vi "TIFF_writeMultipage.vi"(8 "error in":errorcluster, 10 "Array in":T1[](array[typedef]), 11 "file (use dialog)":path=path "D:/TestLV3.tif") -> (0 "error out":errorcluster)   [LabVIEW 2019]
doc: "This VI writes an image array to a multipage tif file. Valid formats are U8 or U16."
uses:
  <vilib>/vision/Image Controls.llb/IMAQ Image.ctl
panel:
  out "First page":T1(plugin-control)
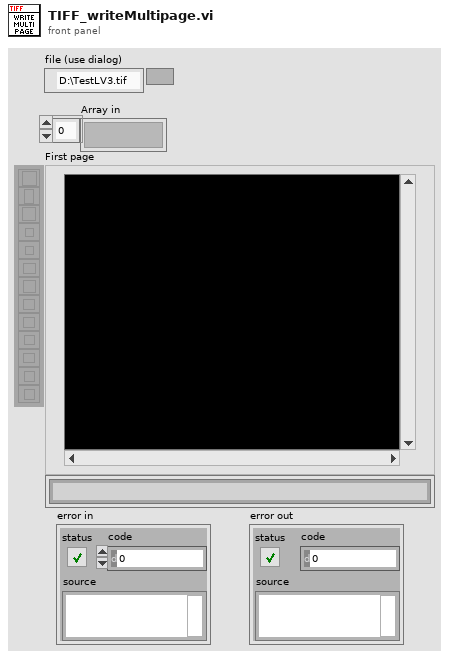
[diagram p1: front panel]
types:
  T1 = typedef "IMAQ Image.ctl" = refnum<image>
  T2 = enum16{"open", "replace", "create", "open or create", "replace or create", "replace or create with confirmation"}
  T3 = enum16{"big-endian, network order", "native, host order", "little-endian"}
  T4 = typedef "Image Type" = u32
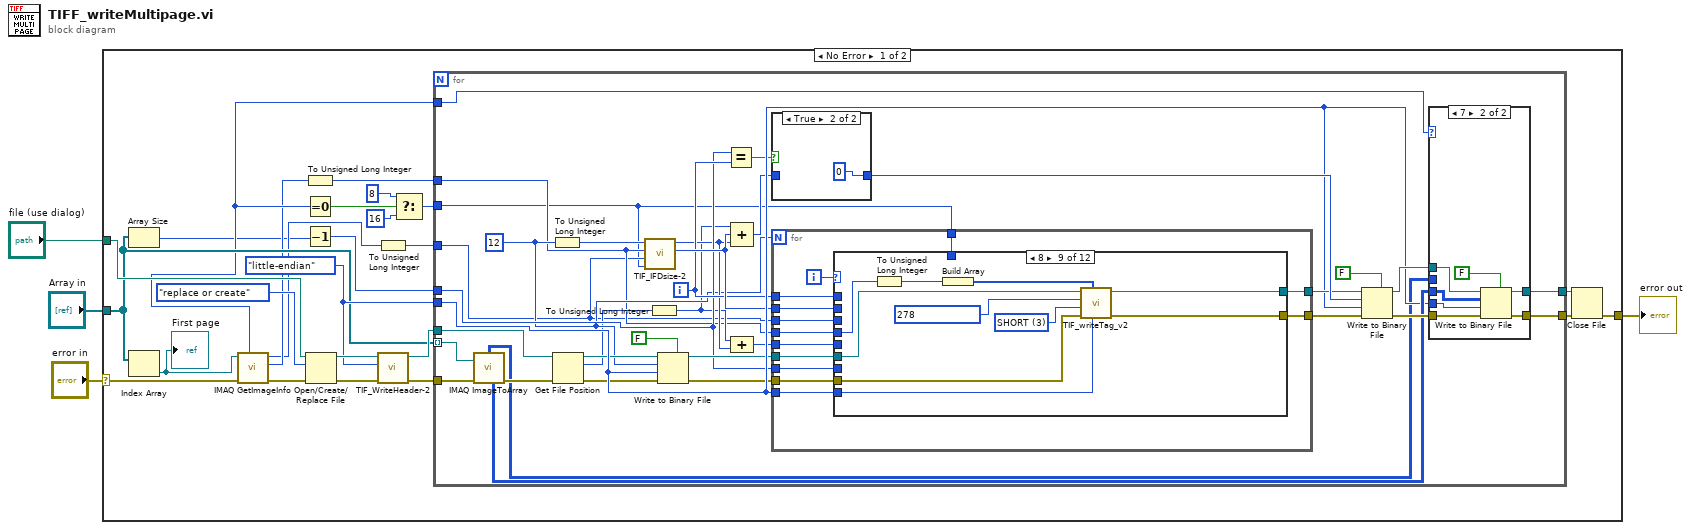
[diagram p0: block diagram]
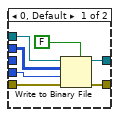
[diagram p2: hidden frame]
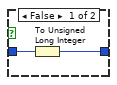
[diagram p3: hidden frame]
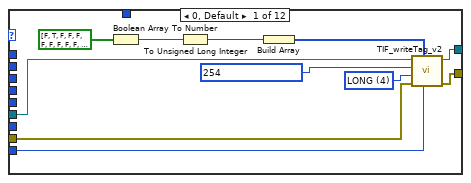
[diagram p4: hidden frame]
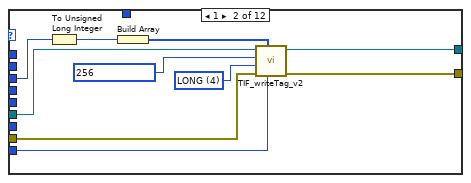
[diagram p5: hidden frame]
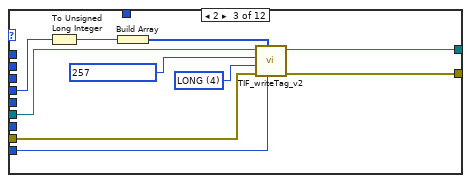
[diagram p6: hidden frame]
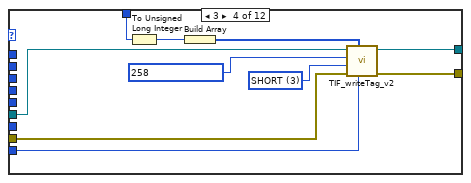
[diagram p7: hidden frame]
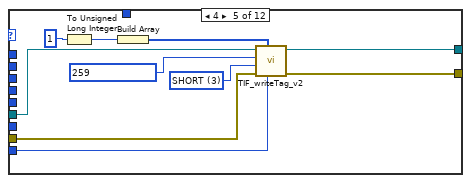
[diagram p8: hidden frame]
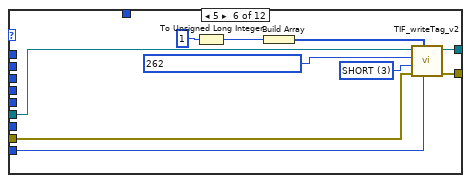
[diagram p9: hidden frame]
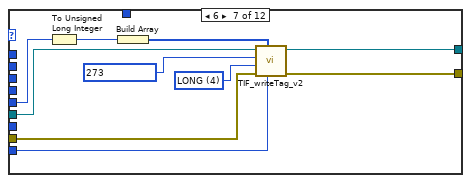
[diagram p10: hidden frame]
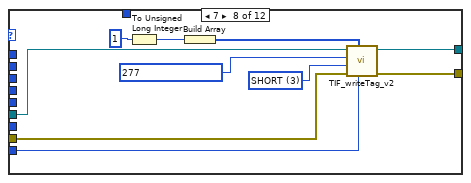
[diagram p11: hidden frame]
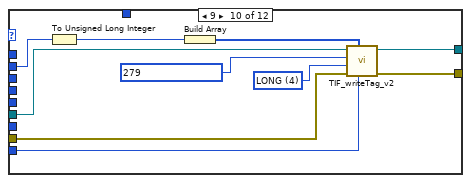
[diagram p12: hidden frame]
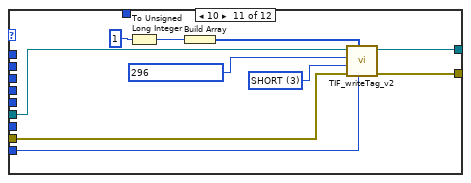
[diagram p13: hidden frame]
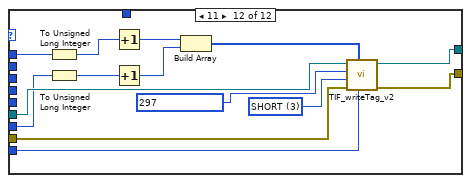
[diagram p14: hidden frame]
diagram:
  n1 = case shown="No Error" "error in" {
    selector: "error in" -> [w16 w220]
    tunnel: "file (use dialog)" -> [w28 _]
    tunnel: "Array in" -> [w22 _]
    tunnel: [w19 w220] -> w1
    frame No Error {
      w26 = T3."little-endian" ("byte order (0:big-endian, network order)")
      n2 = Array Size(array=w22) -> (size(s)=w5:i32)
      n3 = Index Array(array=w22) -> (element=w17:T1)  [unwired: 1 in]
      "First page" <- w17
      n4 = call "IMAQ GetImageInfo"("error in (no error)"=w16, "Image"=w17) -> ("error out"=w15:errorcluster, "Y Resolution"=w7:i32, "X Resolution"=w6:i32, "Image Type"=w11:T4)  [unwired: 2 in, 4 out]
      n5 = To Unsigned Long Integer(number=w7) -> (unsigned 32bit integer=w14:u32)
      n6 = Equal To 0?(x=w11) -> (x = 0?=w12:bool)
      n7 = Decrement(x=w5) -> (x-1=w23:i32)
      n8 = Open/Create/Replace File(file path (use dialog)=w28, error in=w15, operation (0:open)=T2."replace or create") -> (refnum out=w27:refnum<file>, error out=w18:errorcluster)  [unwired: 3 in, 1 out]
      n9 = To Unsigned Long Integer(number=w6) -> (unsigned 32bit integer=w13:u32)
      n10 = call "TIF_WriteHeader-2.vi"("error in"=w18, "[IN] byte order"=w26, "[IN] refnum"=w27) -> ("error out"=w24:errorcluster, "[OUT] refnum"=w25:refnum<file>)  [unwired: 7 in]
      n11 = Select(t=u32 8 ("Bits per sample"), s=w12, f=u32 16 ("Bits per sample")) -> (s? t:f=w8:u32)
      n12 = for {
        tunnel: w22 -> [w64] mode=indexing
        tunnel: w26 -> [w56]
        tunnel: w23 -> [w44]
        tunnel: w25 -> [w52]
        tunnel: w24 -> [w37]
        tunnel: [w38] -> w21
        tunnel: [w30] -> w20
        tunnel: w14 -> [w35]
        tunnel: w13 -> [w34]
        tunnel: w11 -> [w33]
        tunnel: w8 -> [w31]
        i -> [w45]
        w42 = u16 12
        n13 = call "IMAQ ImageToArray"("error in (no error)"=w37, "Image"=w64) -> ("Image Pixels (U16)"=w57:u16[][], "error out"=w36:errorcluster, "Image Pixels (U8)"=w32:u8[][])  [unwired: 2 in, 2 out]
        n14 = To Unsigned Long Integer(number=w42) -> (unsigned 32bit integer=w41:u32)
        n15 = Get File Position(4:w36, 7:w52) -> (0:w50:errorcluster, 2:w40:i64, 3:w51:refnum<file>)
        n16 = call "TIF_IFDsize-2.vi"("[IN] Bits per sample"=w31, "[IN] Image length"=w34, "[IN] Image width"=w35, "[IN] Tags in IFD"=w41) -> ("[OUT] Image size in bytes"=w47:u32, "[OUT] IFD size in bytes"=w43:u32)  [unwired: 6 in]
        n17 = To Unsigned Long Integer(number=w40) -> (unsigned 32bit integer=w39:u32)
        n18 = Write to Binary File(file (use dialog)=w51, data=w42, error in=w50, 5:FALSE ("prepend array or string size? (T)"), 9:w56) -> (refnum out=w54:refnum<file>, error out=w53:errorcluster)  [unwired: 1 in, 1 out]
        n19 = Equal?(x=w44, y=w45) -> (x = y?=w49:bool)
        n20 = Compound Arithmetic op=ADD(w39, w47, w43) -> (w46:u32)
        n21 = Compound Arithmetic op=ADD(w39, w43) -> (w48:u32)
        n22 = case shown="True" w49 {
          tunnel: [w79 u32 0] -> w63
          tunnel: w46 -> [w80 _]
          frame False {
            n23 = To Unsigned Long Integer(number=w80) -> (unsigned 32bit integer=w79:u32)
          }
          frame True {
          }
        }
        n24 = for {
          N: w42 -> [_]
          tunnel: w54 -> [w93]
          tunnel: w53 -> [w92]
          tunnel: w35 -> [w91]
          tunnel: w34 -> [w90]
          tunnel: [w89] -> w61
          tunnel: [w88] -> w60
          tunnel: w56 -> [w87]
          tunnel: w48 -> [w86]
          tunnel: w47 -> [w85]
          tunnel: w45 -> [w84]
          tunnel: w44 -> [w83]
          tunnel: w31 -> [w82]
          i -> [w94]
          n25 = case shown="8" w94 {
            tunnel: w93 -> [w99 w111 w121 w131 w141 w151 w161 w171 w181 w191 w203 w217]
            tunnel: w92 -> [w97 w110 w120 w130 w140 w150 w160 w170 w180 w190 w202 w216]
            tunnel: w91 -> [_ _ w118 _ _ _ _ _ w176 _ _ _]
            tunnel: w90 -> [_ w108 _ _ _ _ _ _ _ _ _ _]
            tunnel: [w98 w109 w119 w129 w138 w148 w159 w168 w179 w189 w198 w215] -> w89
            tunnel: [w95 w107 w117 w127 w136 w146 w157 w166 w178 w188 w196 w214] -> w88
            tunnel: w87 -> [w96 w106 w116 w128 w137 w147 w158 w167 w177 w187 w197 w213]
            tunnel: w86 -> [_ _ _ _ _ _ w156 _ _ _ _ _]
            tunnel: w85 -> [_ _ _ _ _ _ _ _ _ w186 _ _]
            tunnel: w84 -> [_ _ _ _ _ _ _ _ _ _ _ w210]
            tunnel: w83 -> [_ _ _ _ _ _ _ _ _ _ _ w207]
            tunnel: w82 -> [_ _ _ w126 _ _ _ _ _ _ _ _]
            frame 0, Default {
              w105 = u16 4 items=["BYTE"=1, "ASCII"=2, "SHORT"=3, "LONG"=4, "RATIONAL"=5] ("DataType")
              n26 = Boolean Array To Number(Boolean array=bool[] [FALSE, TRUE, FALSE, FALSE, FALSE, FALSE, FALSE, FALSE, FALSE, FALSE, FALSE, FALSE, FALSE, FALSE, FALSE, FALSE, FALSE, FALSE, FALSE, FALSE, FALSE, FALSE, FALSE, FALSE, FALSE, FALSE, FALSE, FALSE, FALSE, FALSE, FALSE, FALSE]) -> (number=w102:u32)
              n27 = To Unsigned Long Integer(number=w102) -> (unsigned 32bit integer=w101:u32)
              n28 = Build Array(w101) -> (w100:u32[])
              n29 = call "TIF_writeTag_v2.vi"("[IN] Byte order"=w96, "[IN] Data"=w100, "error IN"=w97, "[IN] DataType"=w105, "[IN] TagID"=u16 254 ("BaselineTags"), "[IN] refnum"=w99) -> ("error OUT"=w95:errorcluster, "[OUT] refnum"=w98:refnum<file>)  [unwired: 4 in]
            }
            frame 1 {
              w115 = u16 4 items=["BYTE"=1, "ASCII"=2, "SHORT"=3, "LONG"=4, "RATIONAL"=5] ("DataType")
              n30 = To Unsigned Long Integer(number=w108) -> (unsigned 32bit integer=w113:u32)
              n31 = Build Array(w113) -> (w112:u32[])
              n32 = call "TIF_writeTag_v2.vi"("[IN] Byte order"=w106, "[IN] Data"=w112, "error IN"=w110, "[IN] DataType"=w115, "[IN] TagID"=u16 256 ("BaselineTags"), "[IN] refnum"=w111) -> ("error OUT"=w107:errorcluster, "[OUT] refnum"=w109:refnum<file>)  [unwired: 4 in]
            }
            frame 2 {
              w125 = u16 4 items=["BYTE"=1, "ASCII"=2, "SHORT"=3, "LONG"=4, "RATIONAL"=5] ("DataType")
              n33 = To Unsigned Long Integer(number=w118) -> (unsigned 32bit integer=w123:u32)
              n34 = Build Array(w123) -> (w122:u32[])
              n35 = call "TIF_writeTag_v2.vi"("[IN] Byte order"=w116, "[IN] Data"=w122, "error IN"=w120, "[IN] DataType"=w125, "[IN] TagID"=u16 257 ("BaselineTags"), "[IN] refnum"=w121) -> ("error OUT"=w117:errorcluster, "[OUT] refnum"=w119:refnum<file>)  [unwired: 4 in]
            }
            frame 3 {
              w135 = u16 3 items=["BYTE"=1, "ASCII"=2, "SHORT"=3, "LONG"=4, "RATIONAL"=5] ("DataType")
              n36 = To Unsigned Long Integer(number=w126) -> (unsigned 32bit integer=w133:u32)
              n37 = Build Array(w133) -> (w132:u32[])
              n38 = call "TIF_writeTag_v2.vi"("[IN] Byte order"=w128, "[IN] Data"=w132, "error IN"=w130, "[IN] DataType"=w135, "[IN] TagID"=u16 258 ("BaselineTags"), "[IN] refnum"=w131) -> ("error OUT"=w127:errorcluster, "[OUT] refnum"=w129:refnum<file>)  [unwired: 4 in]
            }
            frame 4 {
              w145 = u16 3 items=["BYTE"=1, "ASCII"=2, "SHORT"=3, "LONG"=4, "RATIONAL"=5] ("DataType")
              n39 = To Unsigned Long Integer(number=u32 1) -> (unsigned 32bit integer=w143:u32)
              n40 = Build Array(w143) -> (w142:u32[])
              n41 = call "TIF_writeTag_v2.vi"("[IN] Byte order"=w137, "[IN] Data"=w142, "error IN"=w140, "[IN] DataType"=w145, "[IN] TagID"=u16 259 ("BaselineTags"), "[IN] refnum"=w141) -> ("error OUT"=w136:errorcluster, "[OUT] refnum"=w138:refnum<file>)  [unwired: 4 in]
            }
            frame 5 {
              w155 = u16 3 items=["BYTE"=1, "ASCII"=2, "SHORT"=3, "LONG"=4, "RATIONAL"=5] ("DataType")
              n42 = To Unsigned Long Integer(number=u32 1) -> (unsigned 32bit integer=w153:u32)
              n43 = Build Array(w153) -> (w152:u32[])
              n44 = call "TIF_writeTag_v2.vi"("[IN] Byte order"=w147, "[IN] Data"=w152, "error IN"=w150, "[IN] DataType"=w155, "[IN] TagID"=u16 262 ("BaselineTags"), "[IN] refnum"=w151) -> ("error OUT"=w146:errorcluster, "[OUT] refnum"=w148:refnum<file>)  [unwired: 4 in]
            }
            frame 6 {
              w165 = u16 4 items=["BYTE"=1, "ASCII"=2, "SHORT"=3, "LONG"=4, "RATIONAL"=5] ("DataType")
              n45 = To Unsigned Long Integer(number=w156) -> (unsigned 32bit integer=w163:u32)
              n46 = Build Array(w163) -> (w162:u32[])
              n47 = call "TIF_writeTag_v2.vi"("[IN] Byte order"=w158, "[IN] Data"=w162, "error IN"=w160, "[IN] DataType"=w165, "[IN] TagID"=u16 273 ("BaselineTags"), "[IN] refnum"=w161) -> ("error OUT"=w157:errorcluster, "[OUT] refnum"=w159:refnum<file>)  [unwired: 4 in]
            }
            frame 7 {
              w175 = u16 3 items=["BYTE"=1, "ASCII"=2, "SHORT"=3, "LONG"=4, "RATIONAL"=5] ("DataType")
              n48 = To Unsigned Long Integer(number=u32 1) -> (unsigned 32bit integer=w173:u32)
              n49 = Build Array(w173) -> (w172:u32[])
              n50 = call "TIF_writeTag_v2.vi"("[IN] Byte order"=w167, "[IN] Data"=w172, "error IN"=w170, "[IN] DataType"=w175, "[IN] TagID"=u16 277 ("BaselineTags"), "[IN] refnum"=w171) -> ("error OUT"=w166:errorcluster, "[OUT] refnum"=w168:refnum<file>)  [unwired: 4 in]
            }
            frame 8 {
              w185 = u16 3 items=["BYTE"=1, "ASCII"=2, "SHORT"=3, "LONG"=4, "RATIONAL"=5] ("DataType")
              n51 = To Unsigned Long Integer(number=w176) -> (unsigned 32bit integer=w183:u32)
              n52 = Build Array(w183) -> (w182:u32[])
              n53 = call "TIF_writeTag_v2.vi"("[IN] Byte order"=w177, "[IN] Data"=w182, "error IN"=w180, "[IN] DataType"=w185, "[IN] TagID"=u16 278 ("BaselineTags"), "[IN] refnum"=w181) -> ("error OUT"=w178:errorcluster, "[OUT] refnum"=w179:refnum<file>)  [unwired: 4 in]
            }
            frame 9 {
              w195 = u16 4 items=["BYTE"=1, "ASCII"=2, "SHORT"=3, "LONG"=4, "RATIONAL"=5] ("DataType")
              n54 = To Unsigned Long Integer(number=w186) -> (unsigned 32bit integer=w193:u32)
              n55 = Build Array(w193) -> (w192:u32[])
              n56 = call "TIF_writeTag_v2.vi"("[IN] Byte order"=w187, "[IN] Data"=w192, "error IN"=w190, "[IN] DataType"=w195, "[IN] TagID"=u16 279 ("BaselineTags"), "[IN] refnum"=w191) -> ("error OUT"=w188:errorcluster, "[OUT] refnum"=w189:refnum<file>)  [unwired: 4 in]
            }
            frame 10 {
              w205 = u16 3 items=["BYTE"=1, "ASCII"=2, "SHORT"=3, "LONG"=4, "RATIONAL"=5] ("DataType")
              n57 = To Unsigned Long Integer(number=u32 1) -> (unsigned 32bit integer=w201:u32)
              n58 = Build Array(w201) -> (w200:u32[])
              n59 = call "TIF_writeTag_v2.vi"("[IN] Byte order"=w197, "[IN] Data"=w200, "error IN"=w202, "[IN] DataType"=w205, "[IN] TagID"=u16 296 ("BaselineTags"), "[IN] refnum"=w203) -> ("error OUT"=w196:errorcluster, "[OUT] refnum"=w198:refnum<file>)  [unwired: 4 in]
            }
            frame 11 {
              w219 = u16 3 items=["BYTE"=1, "ASCII"=2, "SHORT"=3, "LONG"=4, "RATIONAL"=5] ("DataType")
              n60 = To Unsigned Long Integer(number=w210) -> (unsigned 32bit integer=w211:u32)
              n61 = To Unsigned Long Integer(number=w207) -> (unsigned 32bit integer=w208:u32)
              n62 = Increment(x=w211) -> (x+1=w212:u32)
              n63 = Increment(x=w208) -> (x+1=w209:u32)
              n64 = Build Array(w212, w209) -> (w206:u32[])
              n65 = call "TIF_writeTag_v2.vi"("[IN] Byte order"=w213, "[IN] Data"=w206, "error IN"=w216, "[IN] DataType"=w219, "[IN] TagID"=u16 297 ("BaselineTags"), "[IN] refnum"=w217) -> ("error OUT"=w214:errorcluster, "[OUT] refnum"=w215:refnum<file>)  [unwired: 4 in]
            }
          }
        }
        n66 = Write to Binary File(file (use dialog)=w61, data=w63, error in=w60, 5:FALSE ("prepend array or string size? (T)"), 9:w56) -> (refnum out=w59:refnum<file>, error out=w58:errorcluster)  [unwired: 1 in, 1 out]
        n67 = case shown="7" w33 {
          tunnel: w59 -> [w70 w77]
          tunnel: w58 -> [w69 w76]
          tunnel: w57 -> [_ w75]
          tunnel: w56 -> [w68 w74]
          tunnel: [w67 w73] -> w38
          tunnel: [w66 w72] -> w30
          tunnel: w32 -> [w65 _]
          frame 0, Default {
            n68 = Write to Binary File(file (use dialog)=w70, data=w65, error in=w69, 5:FALSE ("prepend array or string size? (T)"), 9:w68) -> (refnum out=w66:refnum<file>, error out=w67:errorcluster)  [unwired: 1 in, 1 out]
          }
          frame 7 {
            n69 = Write to Binary File(file (use dialog)=w77, data=w75, error in=w76, 5:FALSE ("prepend array or string size? (T)"), 9:w74) -> (refnum out=w72:refnum<file>, error out=w73:errorcluster)  [unwired: 1 in, 1 out]
          }
        }
      }
      n70 = Close File(refnum=w20, error in=w21) -> (error out=w19:errorcluster)  [unwired: 1 out]
    }
    frame Error {
    }
  }
  "error out" <- w1
